vi "publish -- init -- 6.vi"(7 "publisher action":T1) -> (0 "request event":refnum<user-event>, 1 "response":refnum<user-event>, 4 "data type":cluster{"a":dbl, "b":dbl, "c":cdb})   [LabVIEW 2018]
uses:
  publisher action.ctl
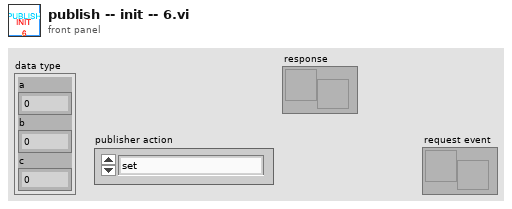
[diagram p1: front panel]
types:
  T1 = typedef "publisher action.ctl" = enum16{"set", "get", "init", "check"}
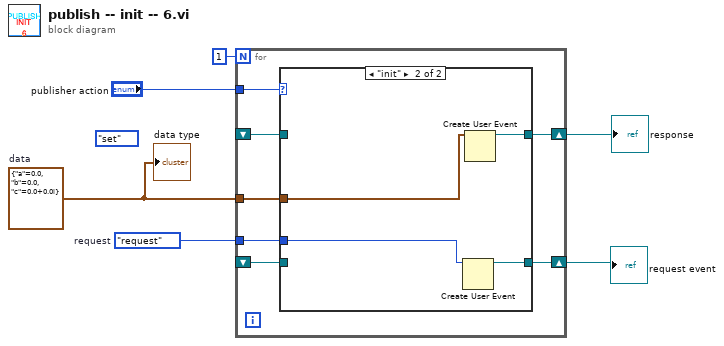
[diagram p0: block diagram]
diagram:
  w1 = cluster{"a":dbl, "b":dbl, "c":cdb} {"a"=0.0, "b"=0.0, "c"=0.0+0.0i}  # data
  w3 = enum16{"request"}."request"  # request
  (unwired) publisher_action."set" ("publisher action")
  n1 = for {
    N: 1 -> [_]
    shift-right: [w13] -> w6
    shift-left: _ -> [w9]
    shift-right: [w12] -> w2
    shift-left: _ -> [w10]
    tunnel: "publisher action" -> [w11]
    tunnel: w1 -> [w8]
    tunnel: w3 -> [w7]
    n2 = case shown="\"init\"" w11 {
      tunnel: [w14 w19] -> w13
      tunnel: [w15 w18] -> w12
      tunnel: w10 -> [w15 _]
      tunnel: w9 -> [w14 _]
      tunnel: w8 -> [_ w17]
      tunnel: w7 -> [_ w16]
      frame "check", Default {
      }
      frame "init" {
        n3 = Create User Event(user event datatype=w16) -> (user event=w19:refnum<user-event>)  [unwired: 1 in, 1 out]
        n4 = Create User Event(user event datatype=w17) -> (user event=w18:refnum<user-event>)  [unwired: 1 in, 1 out]
      }
    }
  }
  "request event" <- w6
  "response" <- w2
  "data type" <- w1
